vi "CloseProject.vi"(11 "Array":string[](array[string])) -> (2 "source":string, 3 "code":i32)   [LabVIEW 2020]
panel:
  out "Error out":errorcluster
  in  "Error_In":errorcluster
  out "path":path
  # "Closes the Project file"
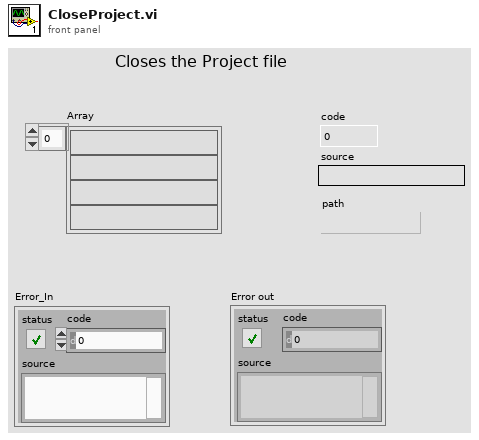
[diagram p1: front panel]
types:
  T1 = enum32{"Invalid", "Standard", "Closed", "Hidden", "Minimized", "Maximized"}
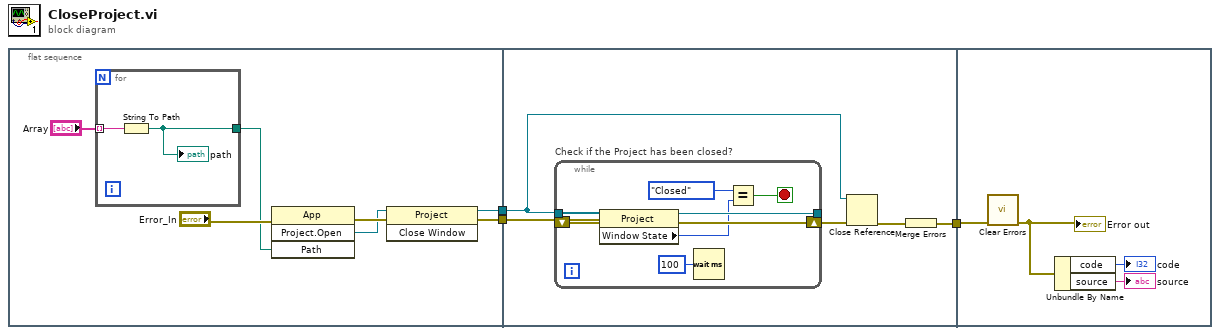
[diagram p0: block diagram]
diagram:
  n1 = flat-sequence {
    tunnel: [w8] -> w3
    tunnel: [w7] -> w2
    tunnel: [w13] -> w1
    tunnel: w3 -> [w15]
    tunnel: w2 -> [w14]
    tunnel: w1 -> [w29]
    frame #0 {
      n2 = for {
        tunnel: [w12] -> w4
        tunnel: "Array" -> [w11] mode=indexing
        n3 = String To Path(string=w11) -> (path=w12:path)
        "path" <- w12
      }
      n4 = invoke class="App" method="Project.Open"(error in="Error_In", "Path"=w4) -> (error out=w10:errorcluster, "Project:Open"=w9:refnum<vi>)  [unwired: 2 in, 2 out]
      n5 = invoke class="Project" method="Close Window"(reference=w9, error in=w10) -> (reference out=w7:refnum<vi>, error out=w8:errorcluster)  [unwired: 1 in, 1 out]
    }
    frame #1 {
      n6 = while "Check if the Project has been closed?" {
        tunnel: [w23] -> _
        shift-right: [w24] -> w16
        shift-left: w15 -> [w19]
        tunnel: w14 -> [w18]
        stop <- w20 stop-if-true
        n7 = property class="Project"(reference=w18, error in=w19) -> (reference out=w23:refnum<vi>, error out=w24:errorcluster, "Window State"=w22:T1)
        n8 = Wait (ms)(milliseconds to wait=u32 100) -> ()  [unwired: 1 out]
        n9 = Equal?(x=T1."Closed" ("Window State 2"), y=w22) -> (x = y?=w20:bool)
      }
      n10 = Close Reference(reference=w14, error in (no error)=w16) -> (error out=w17:errorcluster)
      n11 = Merge Errors(w17) -> (w13:errorcluster)
    }
    frame #2 {
      n12 = call <vilib>:"Clear Errors.vi"("error in (no error)"=w29) -> ("error out"=w28:errorcluster)  [unwired: 5 in, 1 out]
      "Error out" <- w28
      n13 = Unbundle By Name(w28) -> ("code"=→"code":i32, "source"=→"source":string)
    }
  }
